vi "Write Filter.vi"(9 "Filter":string, 11 "CItemMatch in":refnum<class "CItemMatch.lvclass">) -> (3 "CItemMatch out":refnum<class "CItemMatch.lvclass">)   [LabVIEW 2020, in "DependencyInspection.lvlib" / "CItemMatch.lvclass"]
uses:
  CItemMatch.lvclass
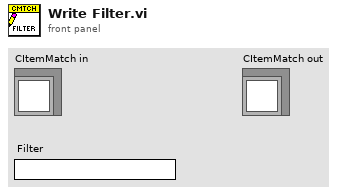
[diagram p1: front panel]
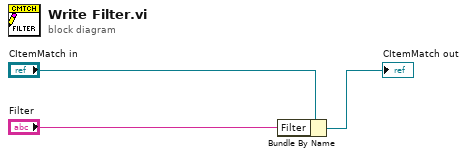
[diagram p0: block diagram]
diagram:
  n1 = Bundle By Name(cluster="CItemMatch in", "Filter"="Filter") -> (→"CItemMatch out":refnum<class "CItemMatch.lvclass">)
